vi "draw.e.vi"(11 "midi-ui in":refnum<class "midi-ui.lvclass">) -> (2 "coordinates":cluster{"x":dbl, "y":dbl}[](array[cluster]), 3 "midi-ui out":refnum<class "midi-ui.lvclass">)   [LabVIEW 2020, in "midi-ui.lvclass"]
uses:
  midi-ui.lvclass
  midi-ui.lvclass/midi-ui.ctl
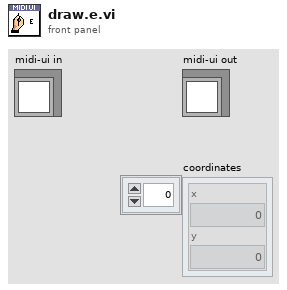
[diagram p1: front panel]
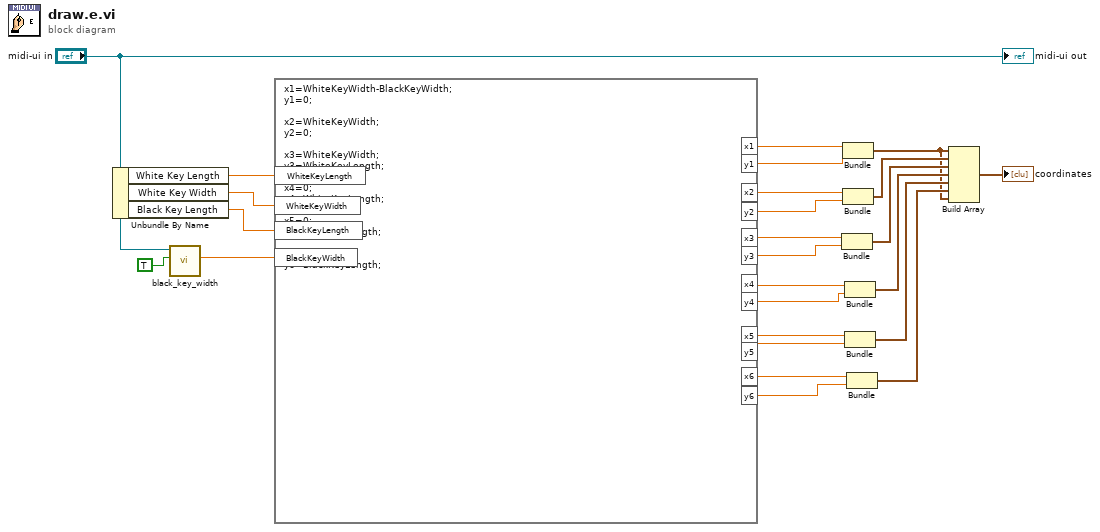
[diagram p0: block diagram]
diagram:
  n1 = Unbundle By Name("midi-ui in") -> ("White Key Length"=w5:dbl, "White Key Width"=w6:dbl, "Black Key Length"=w7:dbl)
  n2 = call "black_key_width.vi"("C# or D#?"=TRUE, "midi-ui in"="midi-ui in") -> ("Black Key Width"=w1:dbl)  [unwired: 8 in, 1 out]
  n3 = formula code="x1=WhiteKeyWidth-BlackKeyWidth;\ny1=0;\n\nx2=WhiteKeyWidth;\ny2=0;\n\nx3=WhiteKeyWidth;\ny3=WhiteKeyLength;\n\nx4=0;\ny4=WhiteKeyLength;\n\nx5=0;\ny5=BlackKeyLength;\n\nx6=x1;\ny6=BlackKeyLength;"("WhiteKeyLength"=w5, "WhiteKeyWidth"=w6, "BlackKeyLength"=w7, "BlackKeyWidth"=w1) -> ("x1"=w25:dbl, "y1"=w24:dbl, "x2"=w16:dbl, "y2"=w17:dbl, "x3"=w18:dbl, "y3"=w23:dbl, "x4"=w19:dbl, "y4"=w20:dbl, "x6"=w21:dbl, "y6"=w22:dbl, "x5"=w10:dbl, "y5"=w11:dbl)
  n4 = Bundle("x3"=w18, "y3"=w23) -> (w14:cluster{"x3":dbl, "y3":dbl})  [unwired: 1 in]
  n5 = Bundle("x1"=w25, "y1"=w24) -> (w4:cluster{"x1":dbl, "y1":dbl})  [unwired: 1 in]
  n6 = Bundle("x2"=w16, "y2"=w17) -> (w15:cluster{"x2":dbl, "y2":dbl})  [unwired: 1 in]
  n7 = Bundle("x4"=w19, "y4"=w20) -> (w13:cluster{"x4":dbl, "y4":dbl})  [unwired: 1 in]
  n8 = Bundle("x5"=w10, "y5"=w11) -> (w9:cluster{"x5":dbl, "y5":dbl})  [unwired: 1 in]
  n9 = Bundle("x6"=w21, "y6"=w22) -> (w12:cluster{"x6":dbl, "y6":dbl})  [unwired: 1 in]
  n10 = Build Array(w4, w15, w14, w13, w9, w12, w4) -> (→"coordinates":cluster{"x1":dbl, "y1":dbl}[])
  "midi-ui out" <- "midi-ui in"
